vi "Build Tree Items Helper.vi"(4 "is array element?":bool, 6 "index string":string, 8 "error in (no error)":errorcluster, 9 "parents":string[](array[string]), 10 "Variant":variant, 11 "Items":T1(array[cluster])) -> (0 "error out":errorcluster, 3 "Items out":T1(array[cluster]))   [LabVIEW 2017, in "Advanced Variant Tools.lvlib"]
uses:
  Advanced Variant Tools.lvlib
  <vilib>/National Instruments/Variant Data Manipulation/Variant Data Manipulation.lvlib
  <vilib>/Utility/Data Type/NI_Data Type.lvlib
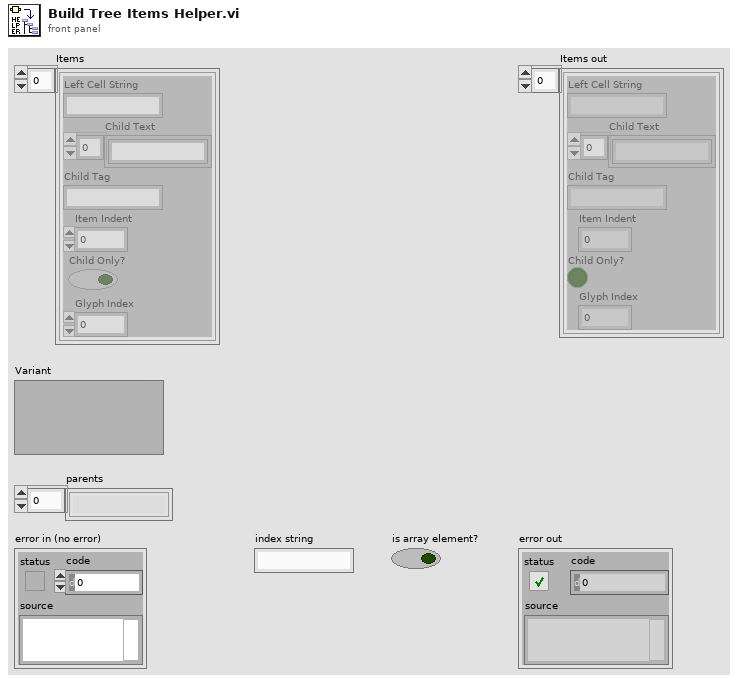
[diagram p1: front panel]
types:
  T1 = cluster{"Left Cell String":string, "Child Text":string[], "Child Tag":string, "Item Indent":i32, "Child Only?":bool, "Glyph Index":i32}[]
  T2 = typedef "NI_Data Type.lvlib/Data Type.ctl" = enum8{"Invalid Type", "Void", "I8", "I16", "I32", "I64", "U8", "U16", "U32", "U64", "Single Float", "Double Float", "Extended Float", "Single Complex", "Double Complex", "Extended Complex", "Enum U8", "Enum U16", "Enum U32", "Enum U64", "Single Float With Unit", "Double Float With Unit", "Extended Float With Unit", "Single Complex with Unit", "Double Complex with Unit", "Extended Complex with Unit", "Boolean", "String", "Path", "Picture", "Tag", "Array", "Cluster", "Variant", "LV Variant", "Waveform", "Timestamp", "Digital Waveform", "Digital Data", "ExpressData", "Refnum", "External Data", "VI", "Poly VI", "LabVIEW Class Instance", "Fixed Point"}
  T3 = cluster{"Left Cell String":string, "Child Text":string[], "Child Tag":string, "Item Indent":i32, "Child Only?":bool, "Glyph Index":i32}
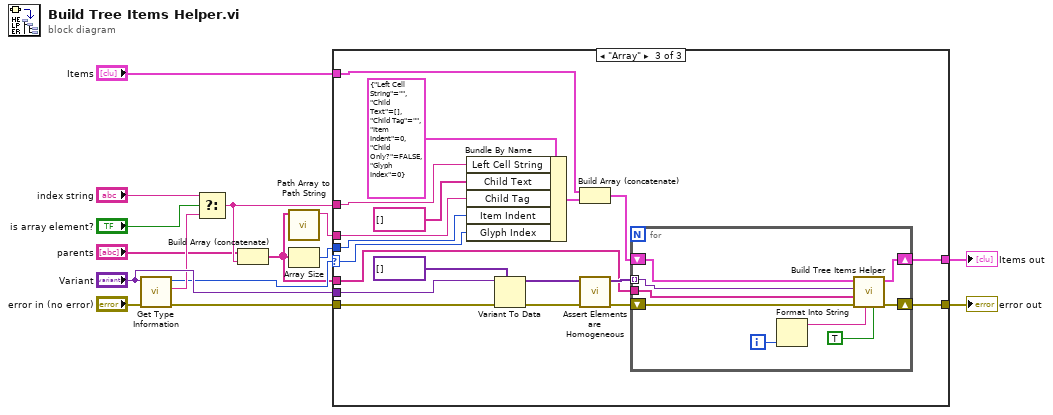
[diagram p0: block diagram]
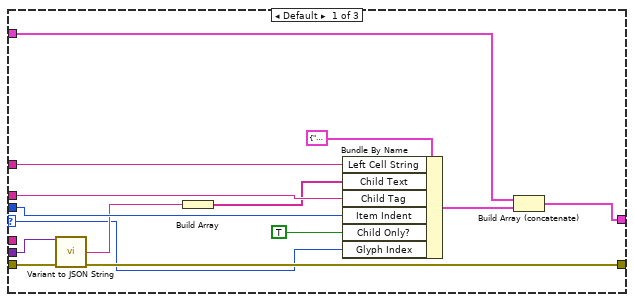
[diagram p2: hidden frame]
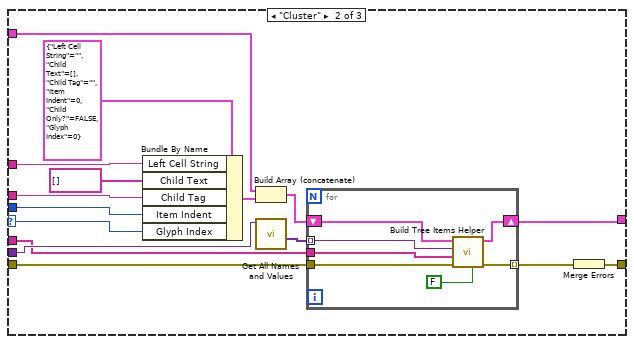
[diagram p3: hidden frame]
diagram:
  n1 = call <vilib>:"Get Type Information.vi"("error in (no error)"="error in (no error)", "Variant"="Variant") -> ("error out"=w15:errorcluster, "Name"=w8:string, "Type"=w5:T2)  [unwired: 5 in, 2 out]
  n2 = Select(t="index string", s="is array element?", f=w8) -> (s? t:f=w6:string)
  n3 = Build Array (concatenate)("parents", w6) -> (w1:string[])
  n4 = call <vilib>:"Path Array to Path String.vi"("path array"=w1) -> ("path"=w4:string)  [unwired: 10 in]
  n5 = Array Size(array=w1) -> (size(s)=w2:i32)
  n6 = case shown="\"Array\"" w5 {
    selector: w5 -> [w16 w30 w53]
    tunnel: w15 -> [w21 w34 w67]
    tunnel: [w20 w42 w71] -> w7
    tunnel: "Variant" -> [w22 w45 w69]
    tunnel: "Items" -> [w29 w41 w61]
    tunnel: [w25 w35 w64] -> w11
    tunnel: w6 -> [w17 w33 w58]
    tunnel: w2 -> [w24 w36 w56]
    tunnel: w4 -> [w23 w37 w57]
    tunnel: w1 -> [_ w32 w55]
    frame Default {
      n7 = call "Variant to JSON String.vi"("Variant in"=w22, "error in (no error)"=w21) -> ("String"=w19:string, "error out"=w20:errorcluster)  [unwired: 11 in, 1 out]
      n8 = Build Array(w19) -> (w18:string[])
      n9 = Bundle By Name(cluster=T3 {"Left Cell String"="", "Child Text"=[], "Child Tag"="", "Item Indent"=0, "Child Only?"=FALSE, "Glyph Index"=0} ("element"), "Left Cell String"=w17, "Child Text"=w18, "Child Tag"=w23, "Item Indent"=w24, "Child Only?"=TRUE, "Glyph Index"=w16) -> (w27:T3)
      n10 = Build Array (concatenate)(w29, w27) -> (w25:T1)
    }
    frame "Cluster" {
      n11 = Bundle By Name(cluster=T3 {"Left Cell String"="", "Child Text"=[], "Child Tag"="", "Item Indent"=0, "Child Only?"=FALSE, "Glyph Index"=0} ("Items"), "Left Cell String"=w33, "Child Text"=string[] [], "Child Tag"=w37, "Item Indent"=w36, "Glyph Index"=w30) -> (w38:T3)
      n12 = Build Array (concatenate)(w41, w38) -> (w39:T1)
      n13 = call <vilib>:"Get All Names and Values.vi"("Cluster in"=w45) -> ("Values"=w44:variant[])  [unwired: 6 in, 4 out]
      n14 = for {
        tunnel: w44 -> [w52] mode=indexing
        tunnel: [w51] -> w43 mode=indexing
        shift-right: [w48] -> w35
        shift-left: w39 -> [w49]
        tunnel: w34 -> [w47]
        tunnel: w32 -> [w46]
        n15 = call "Build Tree Items Helper.vi"("is array element?"=FALSE ("first call?"), "error in (no error)"=w47, "parents"=w46, "Variant"=w52, "Items"=w49) -> ("error out"=w51:errorcluster, "Items out"=w48:T1)  [unwired: 5 in]
      }
      n16 = Merge Errors(w43) -> (w42:errorcluster)
    }
    frame "Array" {
      n17 = Bundle By Name(cluster=T3 {"Left Cell String"="", "Child Text"=[], "Child Tag"="", "Item Indent"=0, "Child Only?"=FALSE, "Glyph Index"=0} ("Items"), "Left Cell String"=w58, "Child Text"=string[] [], "Child Tag"=w57, "Item Indent"=w56, "Glyph Index"=w53) -> (w60:T3)
      n18 = Variant To Data(error in=w67, type=variant[] [], Variant=w69) -> (data=w68:variant[], error out=w66:errorcluster)
      n19 = Build Array (concatenate)(w61, w60) -> (w59:T1)
      n20 = call "Assert Elements are Homogeneous.vi"("error in (no error)"=w66, "array in"=w68) -> ("error out"=w63:errorcluster, "array out"=w65:variant[])  [unwired: 8 in]
      n21 = for {
        tunnel: w65 -> [w77] mode=indexing
        shift-right: [w80] -> w71
        shift-left: w63 -> [w79]
        shift-right: [w75] -> w64
        shift-left: w59 -> [w76]
        tunnel: w55 -> [w72]
        i -> [w74]
        n22 = Format Into String(w74) -> (resulting string=w73:string)  [unwired: 3 in, 1 out]
        n23 = call "Build Tree Items Helper.vi"("is array element?"=TRUE ("first call?"), "index string"=w73, "error in (no error)"=w79, "parents"=w72, "Variant"=w77, "Items"=w76) -> ("error out"=w80:errorcluster, "Items out"=w75:T1)  [unwired: 4 in]
      }
    }
  }
  "Items out" <- w11
  "error out" <- w7
